vi "fg.vi"(5 "action":T1, 7 "section":string[](array[string]), 8 "error in (no error)":errorcluster, 9 "value in":string, 10 "key":string[](array[string]), 11 "path in":path) -> (0 "error out":errorcluster, 1 "value out":string, 2 "exists?":bool, 3 "paths":path[](array[path]))   [LabVIEW 2017, in "toml.lvlib"]
uses:
  toml.lvlib
  fg_action.ctl
  fg_file.ctl
  fg_section.ctl
  fg_row.ctl
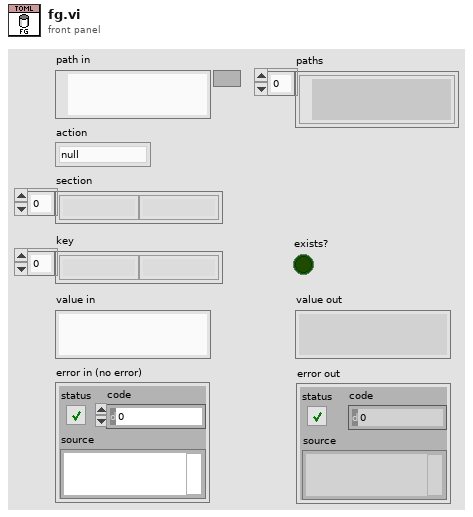
[diagram p1: front panel]
types:
  T1 = typedef "toml.lvlib/fg_action.ctl" = enum8{"null", "get", "set", "pop", "import", "export", "drop", "sections", "keys", "remove"}
  T2 = typedef "toml.lvlib/fg_file.ctl" = cluster{"dirty":bool, "sections":T3[]}
  T3 = typedef "toml.lvlib/fg_section.ctl" = cluster{"section":string[], "rows":T4[], "comment":string}
  T4 = typedef "toml.lvlib/fg_row.ctl" = cluster{"key":string[], "value":string, "comment":string}
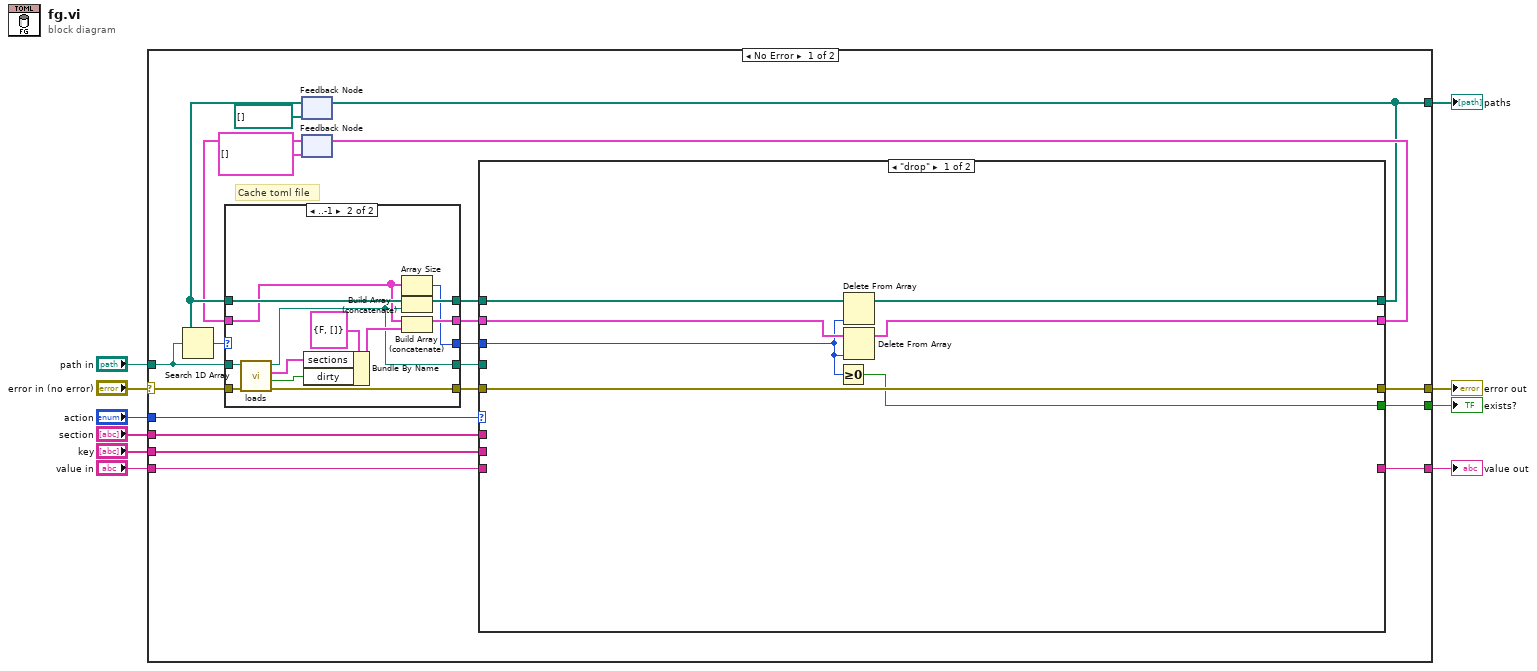
[diagram p0: block diagram]
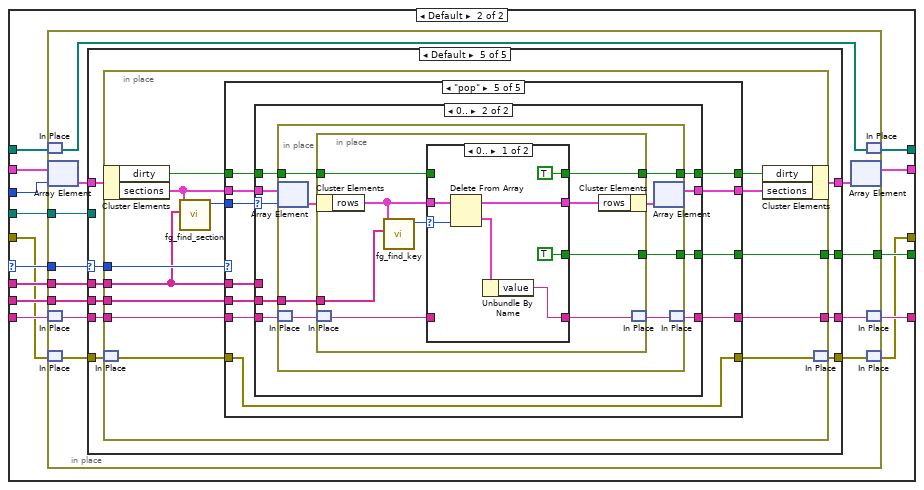
[diagram p2: hidden frame]
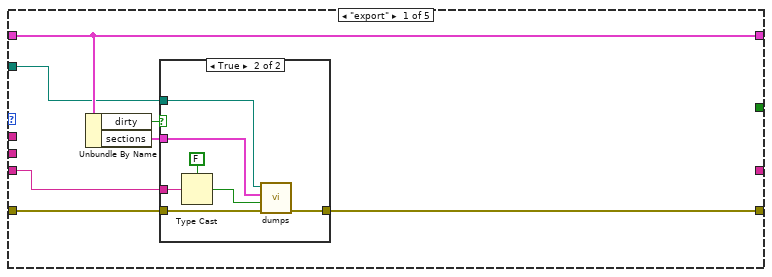
[diagram p3: hidden frame]
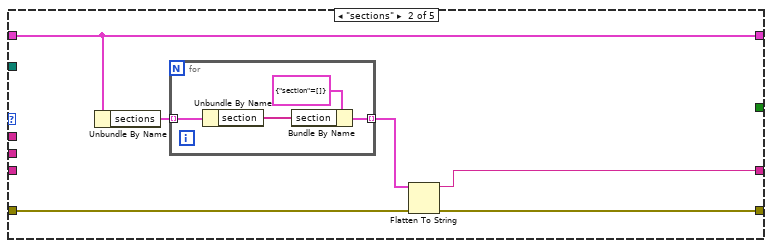
[diagram p5: hidden frame]
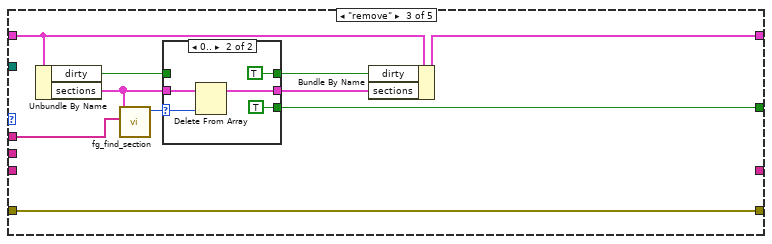
[diagram p6: hidden frame]
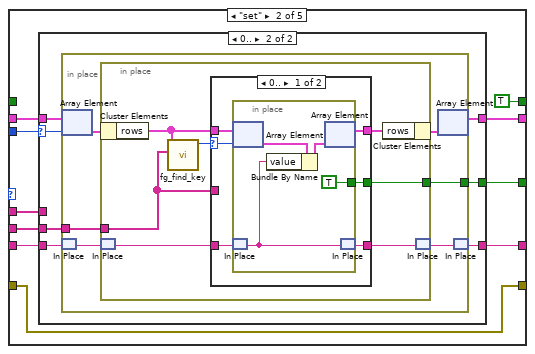
[diagram p10: hidden frame]
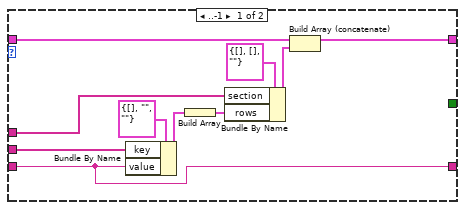
[diagram p11: hidden frame]
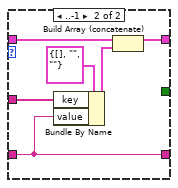
[diagram p12: hidden frame]
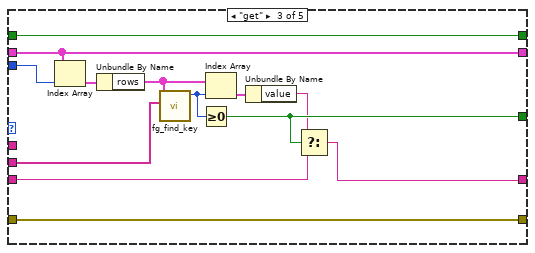
[diagram p13: hidden frame]
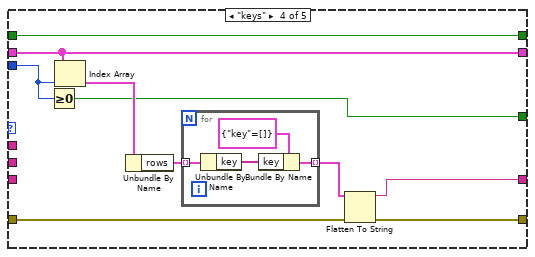
[diagram p14: hidden frame]
diagram:
  n1 = case shown="No Error" "error in (no error)" {
    selector: "error in (no error)" -> [w25 w288]
    tunnel: [w11 _] -> w10
    tunnel: "path in" -> [w26 _]
    tunnel: [w13 w288] -> w7
    tunnel: "action" -> [w19 _]
    tunnel: "section" -> [w22 _]
    tunnel: "key" -> [w20 _]
    tunnel: "value in" -> [w16 w287]
    tunnel: [w18 _] -> w2
    tunnel: [w15 w287] -> w1
    frame No Error {
      # "Cache toml file"
      n2 = feedback #1(path[] []) -> (w28:path[])
      n3 = Search 1D Array(1D array=w28, element=w26) -> (index of element=w29:i32)  [unwired: 1 in]
      n4 = feedback #2(T2[] [] ("files")) -> (w27:T2[])
      n5 = case shown="..-1" w29 {
        selector: w29 -> [w270 _]
        tunnel: w28 -> [w273 w277]
        tunnel: [w273 w286] -> w12
        tunnel: [w272 w285] -> w23
        tunnel: w27 -> [w272 w276]
        tunnel: w26 -> [w269 w284]
        tunnel: [w271 w282] -> w14
        tunnel: w25 -> [w271 w283]
        tunnel: [w270 w281] -> w21
        tunnel: [w269 w274] -> w17
        frame 0.. {
        }
        frame ..-1 {
          n6 = call "loads.vi"("error in (no error)"=w283, "path in"=w284) -> ("error out"=w282:errorcluster, "dirty?"=w275:bool, "sections"=w278:T3[], "path out"=w274:path)  [unwired: 6 in]
          n7 = Bundle By Name(cluster=T2 {"dirty"=FALSE, "sections"=[]} ("file"), "sections"=w278, "dirty"=w275) -> (w279:T2)
          n8 = Array Size(array=w276) -> (size(s)=w281:i32)
          n9 = Build Array (concatenate)(w277, w274) -> (w286:path[])
          n10 = Build Array (concatenate)(w276, w279) -> (w285:T2[])
        }
      }
      n11 = case shown="\"drop\"" w19 {
        selector: w19 -> [_ w47]
        tunnel: [w34 w52] -> w24
        tunnel: w23 -> [w35 w51]
        tunnel: w22 -> [_ w50]
        tunnel: w21 -> [w33 w49]
        tunnel: w20 -> [_ w48]
        tunnel: [w32 w46] -> w18
        tunnel: w17 -> [_ w45]
        tunnel: w16 -> [_ w44]
        tunnel: [_ w43] -> w15
        tunnel: w14 -> [w38 w42]
        tunnel: [w38 w41] -> w13
        tunnel: w12 -> [w37 w40]
        tunnel: [w36 w39] -> w11
        frame "drop" {
          n12 = Greater Or Equal To 0?(x=w33) -> (x >= 0?=w32:bool)
          n13 = Delete From Array(array=w37, index=w33) -> (array with subset deleted=w36:path[])  [unwired: 1 in, 1 out]
          n14 = Delete From Array(array=w35, index=w33) -> (array with subset deleted=w34:T2[])  [unwired: 1 in, 1 out]
        }
        frame Default {
          n15 = in-place {
            in-place-border: w50 -> [w62]
            in-place-border: w48 -> [w61]
            in-place-border: w47 -> [w60]
            in-place-border: [w59] -> w46
            in-place-border: w45 -> [w58]
            n16 = in-place-match #3(w40) -> (w53:path[])
            n17 = in-place-array #4(w51, w49) -> (w64:T2)
            n18 = in-place-match #5(w44) -> (w57:string)
            n19 = in-place-match #6(w42) -> (w55:errorcluster)
            n20 = case shown="Default" w60 {
              selector: w60 -> [_ _ _ _ w114]
              tunnel: w64 -> [w71 w84 w99 w108 w118]
              tunnel: [w71 w84 w97 w108 w117] -> w63
              tunnel: w62 -> [_ _ w98 _ w116]
              tunnel: w61 -> [_ _ _ _ w115]
              tunnel: w57 -> [w65 _ _ _ w113]
              tunnel: [_ _ w90 _ w112] -> w59
              tunnel: [_ w82 _ _ w111] -> w56
              tunnel: w58 -> [w69 _ _ _ _]
              tunnel: w55 -> [w70 w85 w91 w107 w110]
              tunnel: [w68 w83 w91 w107 w109] -> w54
              frame "export" {
                n21 = Unbundle By Name(w71) -> ("dirty"=w67:bool, "sections"=w66:T3[])
                n22 = case shown="True" w67 {
                  tunnel: w70 -> [w72 w79]
                  tunnel: w69 -> [_ w77]
                  tunnel: [w72 w78] -> w68
                  tunnel: w66 -> [_ w76]
                  tunnel: w65 -> [_ w75]
                  frame False {
                  }
                  frame True {
                    n23 = Type Cast(type=FALSE, x=w75) -> (*(type *) &x=w73:bool)
                    n24 = call "dumps.vi"("error in (no error)"=w79, "remove comments? (F)"=w73, "sections"=w76, "path in"=w77) -> ("error out"=w78:errorcluster)  [unwired: 6 in, 1 out]
                  }
                }
              }
              frame "sections" {
                n25 = Unbundle By Name(w84) -> ("sections"=w81:T3[])
                n26 = for {
                  tunnel: w81 -> [w89] mode=indexing
                  tunnel: [w87] -> w80 mode=indexing
                  n27 = Unbundle By Name(w89) -> ("section"=w88:string[])
                  n28 = Bundle By Name(cluster=cluster{"section":string[]} {"section"=[]} ("section"), "section"=w88) -> (w87:cluster{"section":string[]})
                }
                n29 = Flatten To String(anything=w80, error in (no error)=w85) -> (data string=w82:string, error out=w83:errorcluster)  [unwired: 2 in, 1 out]
              }
              frame "remove" {
                n30 = Unbundle By Name(w99) -> ("dirty"=w92:bool, "sections"=w95:T3[])
                n31 = call "fg_find_section.vi"("section"=w98, "sections"=w95) -> ("index"=w93:i32)  [unwired: 9 in]
                n32 = case shown="0.." w93 {
                  selector: w93 -> [_ w103]
                  tunnel: [w101 TRUE ("dirty")] -> w96
                  tunnel: w95 -> [w100 w105]
                  tunnel: [w100 w104] -> w94
                  tunnel: w92 -> [w101 _]
                  tunnel: [_ TRUE] -> w90
                  frame ..-1 {
                  }
                  frame 0.. {
                    n33 = Delete From Array(array=w105, index=w103) -> (array with subset deleted=w104:T3[])  [unwired: 1 in, 1 out]
                  }
                }
                n34 = Bundle By Name(cluster=w99, "dirty"=w96, "sections"=w94) -> (w97:T2)
              }
              frame "import" {
                # "File already loaded do nothing"
              }
              frame Default {
                n35 = in-place {
                  in-place-border: w116 -> [w125]
                  in-place-border: w115 -> [w129]
                  in-place-border: w114 -> [w127]
                  in-place-border: w113 -> [w124]
                  in-place-border: [w123] -> w112
                  in-place-border: [w121] -> w111
                  n36 = in-place-cluster #7(w118) -> ("dirty"=w126:bool, "sections"=w131:T3[])
                  n37 = in-place-match #8(w110) -> (w120:errorcluster)
                  n38 = call "fg_find_section.vi"("section"=w125, "sections"=w131) -> ("index"=w128:i32)  [unwired: 9 in]
                  n39 = case shown="\"pop\"" w127 {
                    tunnel: [w135 TRUE ("dirty") w199 w212 w222] -> w122
                    tunnel: w131 -> [w134 w145 w200 w213 w229]
                    tunnel: [w134 w144 w200 w213 w228] -> w130
                    tunnel: w129 -> [_ w143 w204 _ w227]
                    tunnel: w128 -> [_ w142 w203 w208 w226]
                    tunnel: w126 -> [w135 _ w199 w212 w223]
                    tunnel: w125 -> [_ w141 _ _ w225]
                    tunnel: w124 -> [w133 w140 w196 _ w221]
                    tunnel: [_ w138 w195 w207 w224] -> w123
                    tunnel: [w133 w137 w193 w209 w220] -> w121
                    tunnel: [w132 w136 w192 w205 w219] -> w119
                    tunnel: w120 -> [w132 w136 w192 w206 w219]
                    frame Default {
                    }
                    frame "set" {
                      n40 = case shown="0.." w142 {
                        selector: w142 -> [_ w159]
                        tunnel: w145 -> [w155 w162]
                        tunnel: [w154 w161] -> w144
                        tunnel: w143 -> [w149 w160]
                        tunnel: w141 -> [w151 _]
                        tunnel: w140 -> [w146 w157]
                        tunnel: [_ w158] -> w138
                        tunnel: [w146 w156] -> w137
                        frame ..-1 {
                          n41 = Bundle By Name(cluster=T4 {"key"=[], "value"="", "comment"=""} ("row"), "key"=w149, "value"=w146) -> (w148:T4)
                          n42 = Build Array(w148) -> (w147:T4[])
                          n43 = Bundle By Name(cluster=T3 {"section"=[], "rows"=[], "comment"=""} ("section"), "section"=w151, "rows"=w147) -> (w152:T3)
                          n44 = Build Array (concatenate)(w155, w152) -> (w154:T3[])
                        }
                        frame 0.. {
                          n45 = in-place {
                            in-place-border: w160 -> [w166]
                            in-place-border: [w165] -> w158
                            n46 = in-place-array #9(w162, w159) -> (w168:T3)
                            n47 = in-place-match #10(w157) -> (w164:string)
                            n48 = in-place {
                              in-place-border: w166 -> [w172]
                              in-place-border: [w171] -> w165
                              n49 = in-place-cluster #11(w168) -> ("rows"=w173:T4[])
                              n50 = in-place-match #12(w164) -> (w170:string)
                              n51 = call "fg_find_key.vi"("key"=w172, "rows"=w173) -> ("index"=w175:i32)  [unwired: 9 in]
                              n52 = case shown="0.." w175 {
                                selector: w175 -> [w179 _]
                                tunnel: [w180 w190] -> w174
                                tunnel: w173 -> [w181 w191]
                                tunnel: w172 -> [_ w187]
                                tunnel: w170 -> [w177 w186]
                                tunnel: [w178 _] -> w171
                                tunnel: [w176 w186] -> w169
                                frame 0.. {
                                n53 = in-place {
                                in-place-border: [TRUE ("exists?")] -> w178
                                n54 = in-place-array #13(w181, w179) -> (w185:T4)
                                n55 = in-place-match #14(w177) -> (w182:string)
                                n56 = Bundle By Name(cluster=w185, "value"=w182) -> (w184:T4)
                                n57 = in-place-array #13(w184) -> (w180:T4[])  [unwired: 1 out]
                                n58 = in-place-match #14(w182) -> (w176:string)
                                }
                                }
                                frame ..-1 {
                                n59 = Bundle By Name(cluster=T4 {"key"=[], "value"="", "comment"=""} ("row"), "key"=w187, "value"=w186) -> (w188:T4)
                                n60 = Build Array (concatenate)(w191, w188) -> (w190:T4[])
                                }
                              }
                              n61 = in-place-cluster #11("rows"=w174) -> (w167:T3)
                              n62 = in-place-match #12(w169) -> (w163:string)
                            }
                            n63 = in-place-array #9(w167) -> (w161:T3[])  [unwired: 1 out]
                            n64 = in-place-match #10(w163) -> (w156:string)
                          }
                        }
                      }
                    }
                    frame "get" {
                      n65 = Index Array(array=w200, index=w203) -> (element=w202:T3)
                      n66 = Unbundle By Name(w202) -> ("rows"=w201:T4[])
                      n67 = call "fg_find_key.vi"("key"=w204, "rows"=w201) -> ("index"=w197:i32)  [unwired: 9 in]
                      n68 = Greater Or Equal To 0?(x=w197) -> (x >= 0?=w195:bool)
                      n69 = Index Array(array=w201, index=w197) -> (element=w198:T4)
                      n70 = Unbundle By Name(w198) -> ("value"=w194:string)
                      n71 = Select(t=w194, s=w195, f=w196) -> (s? t:f=w193:string)
                    }
                    frame "keys" {
                      n72 = Greater Or Equal To 0?(x=w208) -> (x >= 0?=w207:bool)
                      n73 = Index Array(array=w213, index=w208) -> (element=w214:T3)
                      n74 = Unbundle By Name(w214) -> ("rows"=w210:T4[])
                      n75 = for {
                        tunnel: w210 -> [w218] mode=indexing
                        tunnel: [w216] -> w211 mode=indexing
                        n76 = Unbundle By Name(w218) -> ("key"=w217:string[])
                        n77 = Bundle By Name(cluster=cluster{"key":string[]} {"key"=[]} ("key"), "key"=w217) -> (w216:cluster{"key":string[]})
                      }
                      n78 = Flatten To String(anything=w211, error in (no error)=w206) -> (data string=w209:string, error out=w205:errorcluster)  [unwired: 2 in, 1 out]
                    }
                    frame "pop" {
                      n79 = case shown="0.." w226 {
                        selector: w226 -> [_ w238]
                        tunnel: w229 -> [w232 w241]
                        tunnel: [w232 w240] -> w228
                        tunnel: w227 -> [_ w239]
                        tunnel: w225 -> [_ _]
                        tunnel: [_ w237] -> w224
                        tunnel: w223 -> [w231 w236]
                        tunnel: [w231 w235] -> w222
                        tunnel: w221 -> [w230 w234]
                        tunnel: [w230 w233] -> w220
                        frame ..-1 {
                        }
                        frame 0.. {
                          n80 = in-place {
                            in-place-border: w239 -> [w247]
                            in-place-border: [w246] -> w237
                            in-place-border: w236 -> [w245]
                            in-place-border: [w244] -> w235
                            n81 = in-place-array #15(w241, w238) -> (w249:T3)
                            n82 = in-place-match #16(w234) -> (w243:string)
                            n83 = in-place {
                              in-place-border: w247 -> [w255]
                              in-place-border: [w254] -> w246
                              in-place-border: w245 -> [w253]
                              in-place-border: [w252] -> w244
                              n84 = in-place-cluster #17(w249) -> ("rows"=w256:T4[])
                              n85 = in-place-match #18(w243) -> (w251:string)
                              n86 = call "fg_find_key.vi"("key"=w255, "rows"=w256) -> ("index"=w258:i32)  [unwired: 9 in]
                              n87 = case shown="0.." w258 {
                                selector: w258 -> [w263 _]
                                tunnel: [w262 w268] -> w257
                                tunnel: w256 -> [w264 w268]
                                tunnel: [TRUE ("exists?") _] -> w254
                                tunnel: w253 -> [_ w267]
                                tunnel: [TRUE ("exists?") w267] -> w252
                                tunnel: w251 -> [_ w266]
                                tunnel: [w259 w266] -> w250
                                frame 0.. {
                                n88 = Delete From Array(array=w264, index=w263) -> (deleted portion=w260:T4, array with subset deleted=w262:T4[])  [unwired: 1 in]
                                n89 = Unbundle By Name(w260) -> ("value"=w259:string)
                                }
                                frame ..-1 {
                                }
                              }
                              n90 = in-place-cluster #17("rows"=w257) -> (w248:T3)
                              n91 = in-place-match #18(w250) -> (w242:string)
                            }
                            n92 = in-place-array #15(w248) -> (w240:T3[])  [unwired: 1 out]
                            n93 = in-place-match #16(w242) -> (w233:string)
                          }
                        }
                      }
                    }
                  }
                  n94 = in-place-cluster #7("dirty"=w122, "sections"=w130) -> (w117:T2)
                  n95 = in-place-match #8(w119) -> (w109:errorcluster)
                }
              }
            }
            n96 = in-place-array #4(w63) -> (w52:T2[])  [unwired: 1 out]
            n97 = in-place-match #3(w53) -> (w39:path[])
            n98 = in-place-match #5(w56) -> (w43:string)
            n99 = in-place-match #6(w54) -> (w41:errorcluster)
          }
        }
      }
      n100 = feedback-in #1(w11) -> ()
      n101 = feedback-in #2(w24) -> ()
    }
    frame Error {
    }
  }
  "error out" <- w7
  "value out" <- w1
  "exists?" <- w2
  "paths" <- w10
